vi "Analog In Error Counter.vi"(8 "error in (no error)":errorcluster, 9 "Max Errors":i32=1, 10 "Count":i32, 11 "Unit":i32) -> (0 "Fault":bool, 3 "Numeric out":i32)   [LabVIEW 2017]
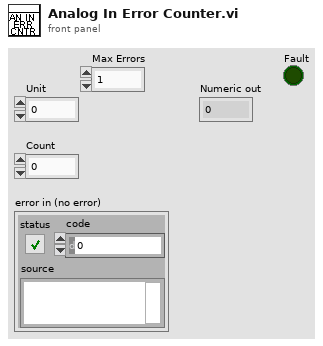
[diagram p1: front panel]
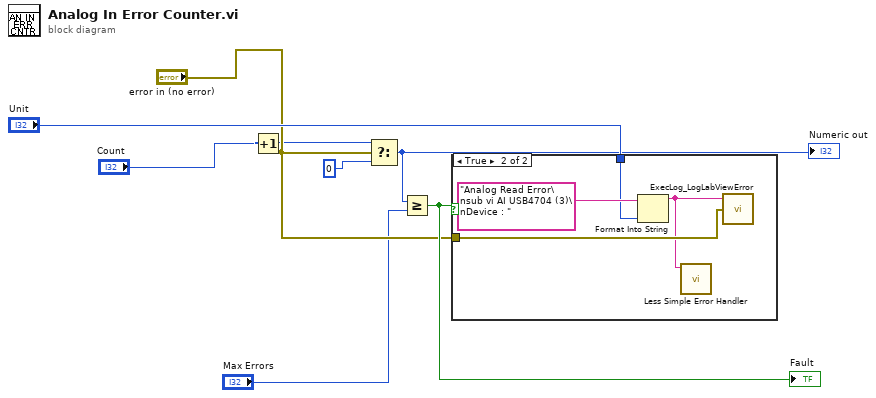
[diagram p0: block diagram]
diagram:
  n1 = Increment(x="Count") -> (x+1=w3:i32)
  n2 = Select(t=w3, s="error in (no error)", f=0) -> (s? t:f=w4:i32)
  "Numeric out" <- w4
  n3 = Greater Or Equal?(x=w4, y="Max Errors") -> (x >= y?=w7:bool)
  "Fault" <- w7
  n4 = case shown="True" w7 {
    tunnel: "error in (no error)" -> [_ w10]
    tunnel: "Unit" -> [_ w11]
    frame False {
    }
    frame True {
      n5 = Format Into String(initial string="Analog Read Error\nsub vi AI USB4704 (3)\nDevice : " ("message"), w11) -> (resulting string=w9:string)  [unwired: 2 in, 1 out]
      n6 = call "Less Simple Error Handler.vi"("message"=w9) -> ()  [unwired: 5 in]
      n7 = call "ExecLog_LogLabViewError.vi"("error IO"=w10, "string 1"=w9) -> ()  [unwired: 2 in, 1 out]
    }
  }
